vi "Page_Source_Initialize.vi"(8 "error in (no error)":errorcluster, 11 "ctlReferences":T1) -> (0 "error out":errorcluster)   [LabVIEW 2020, in "AB_EXE.lvlib"]
uses:
  <vilib>/AppBuilder/AB_Classes/EXE/common/AB_EXE.lvlib
  <resource>/Framework/Providers/Common/provcom_StringGlobals.vi
  <resource>/Framework/Providers/Builds/AppBuilder/AB_UI_Page_Source_Files_References.ctl
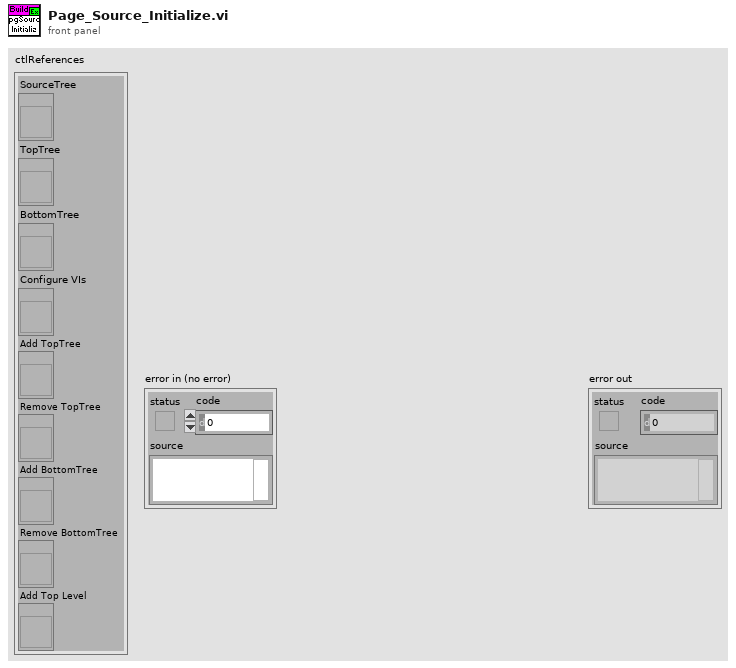
[diagram p1: front panel]
types:
  T1 = typedef "AB_UI_Page_Source_Files_References.ctl" = cluster{"SourceTree":refnum<vi>, "TopTree":refnum<vi>, "BottomTree":refnum<vi>, "Configure VIs":refnum<vi>, "Add TopTree":refnum<vi>, "Remove TopTree":refnum<vi>, "Add BottomTree":refnum<vi>, "Remove BottomTree":refnum<vi>, "Add Top Level":refnum<vi>}
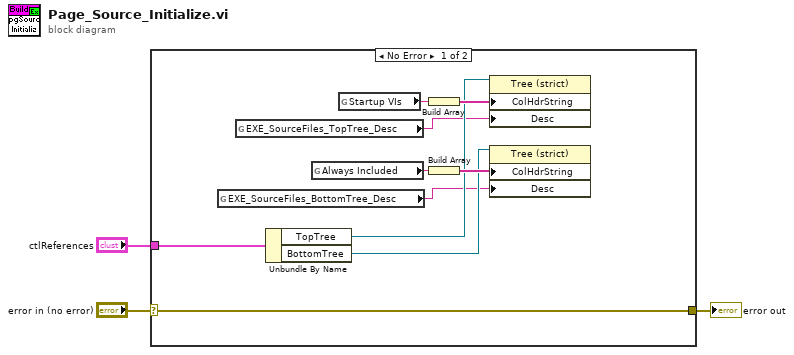
[diagram p0: block diagram]
diagram:
  n1 = case shown="No Error" "error in (no error)" {
    selector: "error in (no error)" -> [w4 w14]
    tunnel: "ctlReferences" -> [w5 _]
    tunnel: [w4 w14] -> w1
    frame No Error {
      n2 = global read "provcom_StringGlobals.vi" "EXE_SourceFiles_BottomTree_Desc"() -> (w6:string)
      n3 = global read "provcom_StringGlobals.vi" "EXE_SourceFiles_TopTree_Desc"() -> (w7:string)
      n4 = Unbundle By Name(w5) -> ("TopTree"=w9:refnum<vi>, "BottomTree"=w8:refnum<vi>)
      n5 = global read "provcom_StringGlobals.vi" "Always Included"() -> (w13:string)
      n6 = global read "provcom_StringGlobals.vi" "Startup VIs"() -> (w12:string)
      n7 = Build Array(w12) -> (w11:string[])
      n8 = Build Array(w13) -> (w10:string[])
      n9 = property class="Tree (strict)"(reference=w9, "ColHdrString"=w11, "Desc"=w7) -> ()  [unwired: 1 in, 2 out]
      n10 = property class="Tree (strict)"(reference=w8, "ColHdrString"=w10, "Desc"=w6) -> ()  [unwired: 1 in, 2 out]
    }
    frame Error {
    }
  }
  "error out" <- w1
